vi "Visual - Read All Data_SubVIs-某型振动实验台测试系统.vi"(8 "error in":errorcluster) -> (0 "error out":errorcluster, 3 "Data":dbl[][](array[numeric]))   [LabVIEW 2009]
doc: "Use this template to build a VI to use as a subVI."
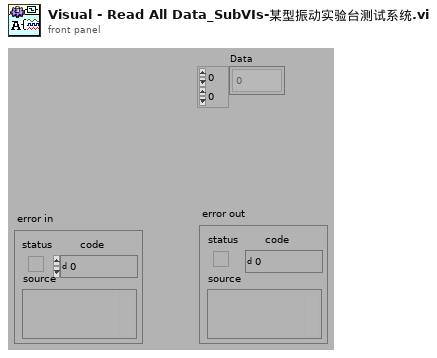
[diagram p1: front panel]
types:
  T1 = enum16{"open", "open or create", "create or replace", "create", "open (read-only)"}
  T2 = enum32{"invalid app kind", "Development System", "Run Time System", "Student Edition", "Embedded LabVIEW", "Evaluation", "Custom"}
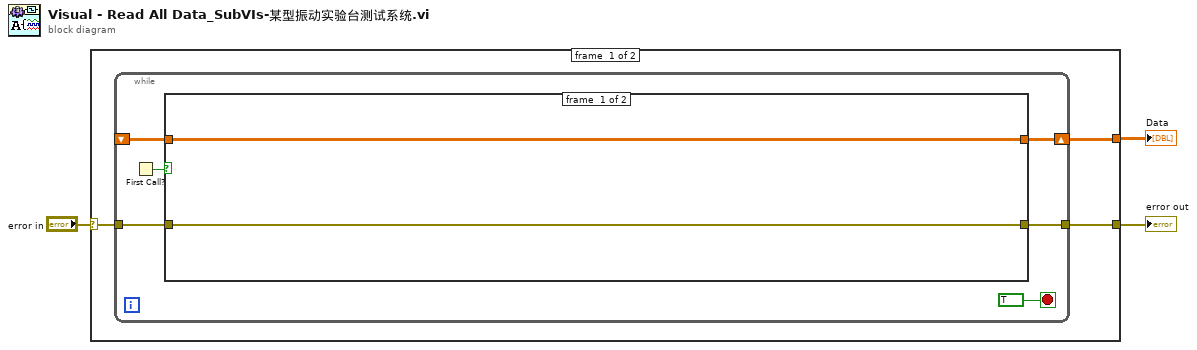
[diagram p0: block diagram]
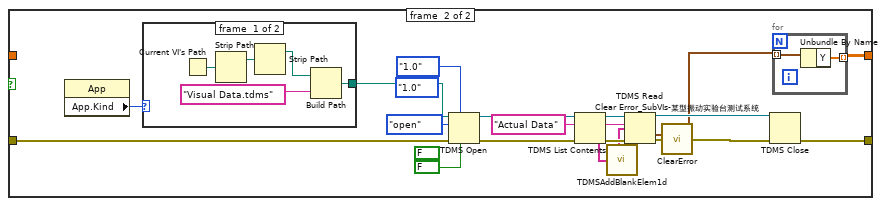
[diagram p2: hidden frame]
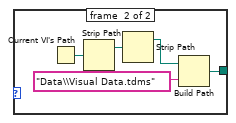
[diagram p3: hidden frame]
diagram:
  n1 = case shown="无错误" "error in" {
    selector: "error in" -> [w6 w48]
    tunnel: [w5 w48] -> w2
    tunnel: [w4 _] -> w1
    frame #0 {
      n2 = while {
        tunnel: w6 -> [w12]
        tunnel: [w11] -> w5
        shift-right: [w10] -> w4
        shift-left: _ -> [w7]
        stop <- TRUE stop-if-true
        n3 = First Call?() -> (First Call?: T/F=w8:bool)
        n4 = case shown="真" w8 {
          tunnel: w12 -> [w13 w35]
          tunnel: [w13 w34] -> w11
          tunnel: [w14 w33] -> w10
          tunnel: w7 -> [w14 _]
          frame #0 {
          }
          frame #1 {
            (unwired) enum16{"1.0", "2.0"}."1.0" ("file format version (2.0)")
            (unwired) FALSE ("disable buffering (T)")
            n5 = property class="App"() -> ("App.Kind"=w22:T2)  [unwired: 2 in, 2 out]
            n6 = case shown="\"Development System\"" w22 {
              tunnel: [w36 w41] -> w21
              frame #0 {
                n7 = Current VI's Path() -> (path=w40:path)
                n8 = Strip Path(path=w40) -> (stripped path=w39:path)  [unwired: 1 out]
                n9 = Strip Path(path=w39) -> (stripped path=w38:path)  [unwired: 1 out]
                n10 = Build Path(base path=w38, name or relative path="Visual Data.tdms") -> (appended path=w36:path)
              }
              frame #1 {
                n11 = Current VI's Path() -> (path=w42:path)
                n12 = Strip Path(path=w42) -> (stripped path=w43:path)  [unwired: 1 out]
                n13 = Strip Path(path=w43) -> (stripped path=w44:path)  [unwired: 1 out]
                n14 = Build Path(base path=w44, name or relative path="Data\\Visual Data.tdms") -> (appended path=w41:path)
              }
            }
            n15 = TDMS Open(6:FALSE ("禁用缓存(T)"), 7:enum16{"1.0", "2.0"}."1.0" ("文件格式版本(2.0)"), 8:w35, 10:T1."open" ("operation (0:open)"), 11:w21) -> (0:w24:errorcluster, 3:w25:refnum<k34>)  [unwired: 1 in]
            n16 = TDMS List Contents(4:w24, 6:"Actual Data" ("group name"), 7:w25) -> (0:w28:errorcluster, 1:w15:string[], 2:w27:string, 3:w29:refnum<k34>)
            n17 = call <vilib>:"TDMSAddBlankElem1d.vi"("input string array"=w15) -> ("output string array with blank element at the beginning"=w19:string[])
            n18 = TDMS Read(0:w29, 5:w27, 7:w19, 11:w28) -> (4:w32:refnum<k34>, 10:w23:waveform(dbl)[], 15:w16:errorcluster)  [unwired: 6 out]
            n19 = call <vilib>:"ClearError.vi"("error in (no error)"=w16) -> ("error out"=w20:errorcluster)
            n20 = call "Clear Error_SubVIs-某型振动实验台测试系统.vi"("error in (no error)"=w20) -> ("error out"=w31:errorcluster)
            n21 = TDMS Close(8:w31, 11:w32) -> (0:w34:errorcluster)
            n22 = for {
              tunnel: w23 -> [w47] mode=indexing
              tunnel: [w46] -> w33 mode=indexing
              n23 = Unbundle By Name(w47) -> ("Y"=w46:dbl[])
            }
          }
        }
      }
    }
    frame #1 {
    }
  }
  "error out" <- w2
  "Data" <- w1
